vi "AWG Configure.vi"(6 "Output Mode":T1=4 caption="Output Mode (default: 0=Standard Function)" items=["Standard Function", "Frequency List", "Arbitrary Waveform", "Arbitrary Sequence", "Script"], 7 "Sample Clock Source":string(combo)="OnboardClock", 8 "error in (no error)":errorcluster, 9 "Sample Rate":dbl=20000000.0 format="%.2p", 10 "Pins":string[](array[string]), 11 "Semiconductor Module Context":T2) -> (0 "error out":errorcluster, 2 "Instrument Sessions Out":refnum<k15>[](array[refnum]), 3 "Semiconductor Module Context Out":T2)   [LabVIEW 2013]
uses:
  <vilib>/NI_TestStand_SemiconductorModule/NI_TestStand_Semiconductor_Module.lvlibp/PinMap/General/SemiconductorModuleContext.ctl
  <instrlib>/niFgen/niFgen.llb/niFgen Output Mode.ctl
  <instrlib>/niFgen/niFgen.llb/niFgen_ctl Trigger Script - trigID Values (Ring).ctl
  <instrlib>/niFgen/niFgen.llb/niFgen Configure Software Edge Script Trigger.vi
  <vilib>/Utility/error.llb/Error Cluster From Error Code.vi
  <vilib>/ErrorRing/Error Ring.xnode
  <vilib>/NI_TestStand_SemiconductorModule/NI_TestStand_Semiconductor_Module.lvlibp
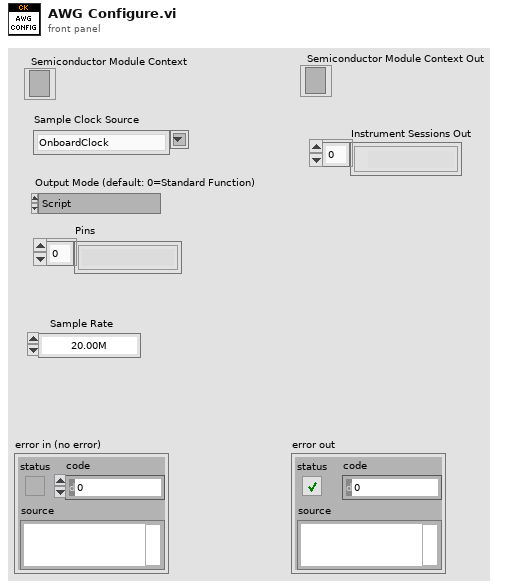
[diagram p1: front panel]
types:
  T1 = typedef "niFgen Output Mode.ctl" = u32
  T2 = typedef "NI_TestStand_Semiconductor_Module.lvlibp/SemiconductorModuleContext.ctl" = refnum<k7>
  T3 = typedef "niFgen_ctl Trigger Script - trigID Values (Ring).ctl" = string
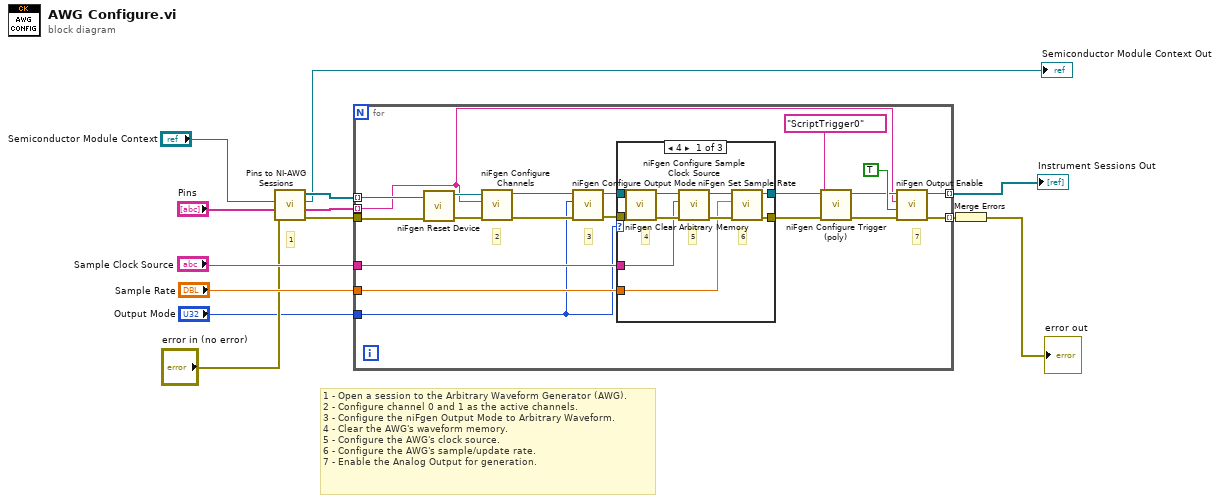
[diagram p0: block diagram]
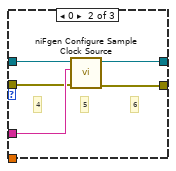
[diagram p2: hidden frame]
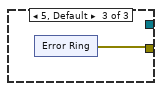
[diagram p3: hidden frame]
diagram:
  # "1"
  # "1 - Open a session to the Arbitrary Waveform Generator (AWG).\n2 - Configure channel 0 and 1 as the active channels.\n3 - Configure the niFgen Output Mode to Arbitrary Waveform.\n4 - Clear the AWG's waveform memory.\n5 - Configure the AWG's clock source.\n6 - Configure the AWG's sample/update rate.\n7 - Enable the Analog Output for generation."
  n1 = call "Pins to NI-AWG Sessions.vi"("error in (no error)"="error in (no error)", "Pins"="Pins", "Semiconductor Module Context"="Semiconductor Module Context") -> ("error out"=w12:errorcluster, "Channel Lists"=w11:string[], "Semiconductor Module Context Out"=→"Semiconductor Module Context Out":T2, "Instrument Sessions"=w13:refnum<k15>[])  [unwired: 5 in]
  n2 = for {
    tunnel: w13 -> [w22] mode=indexing
    tunnel: w12 -> [w23]
    tunnel: w11 -> [w14] mode=indexing
    tunnel: "Sample Clock Source" -> [w28]
    tunnel: "Sample Rate" -> [w27]
    tunnel: [w26] -> w4 mode=indexing
    tunnel: [w25] -> w3 mode=indexing
    tunnel: "Output Mode" -> [w20]
    # "2"
    # "3"
    # "7"
    n3 = call <instrlib>:"niFgen Reset Device.vi"("error in (no error)"=w23, "Instrument Handle"=w22) -> ("error out"=w24:errorcluster, "Instrument Handle Out"=w21:refnum<k15>)  [unwired: 8 in]
    n4 = call <instrlib>:"niFgen Configure Channels.vi"("error in (no error)"=w24, "Channels"=w14, "Instrument Handle"=w21) -> ("error out"=w29:errorcluster, "Instrument Handle Out"=w30:refnum<k15>)  [unwired: 7 in]
    n5 = call <instrlib>:"niFgen Configure Output Mode.vi"("error in (no error)"=w29, "Output Mode (default: 0=Standard Function)"=w20, "Instrument Handle"=w30) -> ("error out"=w32:errorcluster, "Instrument Handle Out"=w33:refnum<k15>)  [unwired: 6 in]
    n6 = case shown="4" w20 {
      tunnel: w33 -> [w43 w47 _]
      tunnel: w32 -> [w42 w46 _]
      tunnel: [w37 w45 _] -> w17
      tunnel: [w36 w44 w49] -> w16
      tunnel: w28 -> [w35 w48 _]
      tunnel: w27 -> [w34 _ _]
      frame 4 {
        # "6"
        # "5"
        # "4"
        n7 = call <instrlib>:"niFgen Clear Arbitrary Memory.vi"("error in (no error)"=w42, "Instrument Handle"=w43) -> ("error out"=w38:errorcluster, "Instrument Handle Out"=w39:refnum<k15>)  [unwired: 8 in]
        n8 = call <instrlib>:"niFgen Configure Sample Clock Source.vi"("error in (no error)"=w38, "Source (Onboard Clock)"=w35, "Instrument Handle"=w39) -> ("error out"=w40:errorcluster, "Instrument Handle Out"=w41:refnum<k15>)  [unwired: 7 in]
        n9 = call <instrlib>:"niFgen Set Sample Rate.vi"("error in (no error)"=w40, "Sample Rate (Samp/s)"=w34, "Instrument Handle"=w41) -> ("error out"=w36:errorcluster, "Instrument Handle Out"=w37:refnum<k15>)  [unwired: 7 in]
      }
      frame 0 {
        # "6"
        # "5"
        # "4"
        n10 = call <instrlib>:"niFgen Configure Sample Clock Source.vi"("error in (no error)"=w46, "Source (Onboard Clock)"=w48, "Instrument Handle"=w47) -> ("error out"=w44:errorcluster, "Instrument Handle Out"=w45:refnum<k15>)  [unwired: 7 in]
      }
      frame 5, Default {
        n11 = xnode "Error Ring"() -> ("error out"=w49:errorcluster)
      }
    }
    n12 = call-poly <instrlib>:"niFgen Configure Trigger (poly).vi"("error in (no error)"=w16, "Trigger ID (Script Trigger 0)"=T3 "ScriptTrigger0", "Instrument Handle"=w17) -> ("error out"=w19:errorcluster, "Instrument Handle Out"=w18:refnum<k15>)  [unwired: 7 in]
    n13 = call <instrlib>:"niFgen Output Enable.vi"("error in (no error)"=w19, "Output Enable (default: True)"=TRUE ("output enable"), "Channel Name"=w14, "Instrument Handle"=w18) -> ("error out"=w26:errorcluster, "Instrument Handle Out"=w25:refnum<k15>)  [unwired: 6 in]
  }
  "Instrument Sessions Out" <- w3
  n14 = Merge Errors(w4) -> (→"error out":errorcluster)
